vi "GUNSC_verifyNumExtensions.vi"(8 "current_extensions":u16[](array[numeric]), 9 "geom_num_amplif":i32) -> (1 "current_extensions out":u16[](array[numeric]))   [LabVIEW 2014]
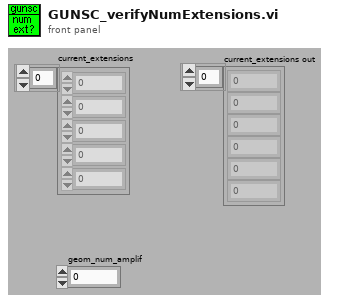
[diagram p1: front panel]
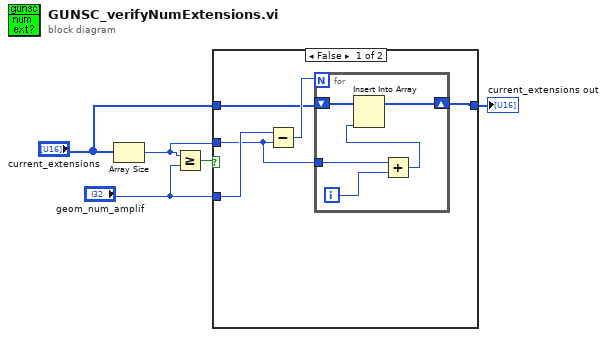
[diagram p0: block diagram]
diagram:
  n1 = Array Size(array="current_extensions") -> (size(s)=w1:i32)
  n2 = Greater Or Equal?(x=w1, y="geom_num_amplif") -> (x >= y?=w5:bool)
  n3 = case shown="False" w5 {
    tunnel: "current_extensions" -> [w8 w16]
    tunnel: [w6 w16] -> w3
    tunnel: "geom_num_amplif" -> [w10 _]
    tunnel: w1 -> [w7 _]
    frame False {
      n4 = Subtract(x=w10, y=w7) -> (x-y=w9:i32)
      n5 = for {
        N: w9 -> [_]
        shift-right: [w12] -> w6
        shift-left: w8 -> [w15]
        tunnel: w7 -> [w14]
        i -> [w11]
        n6 = Add(x=w14, y=w11) -> (x+y=w13:i32)
        n7 = Insert Into Array(array=w15, new element=w13) -> (w12:u16[])  [unwired: 1 in]
      }
    }
    frame True {
    }
  }
  "current_extensions out" <- w3
